vi "Lift main.vi"() -> ()   [LabVIEW 2018]
uses:
  <vilib>/Rock Robotics/WPI/ThirdParty/Phoenix-LabVIEW/Motor Controller/Controls/CTRE_Phoenix_MotorControl_FeedbackDevice.ctl
  <vilib>/Rock Robotics/WPI/ThirdParty/Phoenix-LabVIEW/Motor Controller/Controls/CTRE_Phoenix_MotorControl_ControlMode.ctl
  <vilib>/Rock Robotics/WPI/ThirdParty/Phoenix-LabVIEW/Motor Controller/Get/CTRE_Phoenix_MotorController_GetSelectedSensorData.vi
  <vilib>/Rock Robotics/Network Tables/NT Write Number.vi
  <vilib>/Rock Robotics/Network Tables/NT Read Boolean.vi
  Robot Global Data.vi
  <vilib>/Rock Robotics/Network Tables/NT Read Number.vi
  <vilib>/Rock Robotics/WPI/Solenoid/Deprecated/WPI_SolenoidSetBool.vi
panel:
  in  "Calibrate Lift":bool
  in  "Lift Setpoint":dbl
  in  "Enable Manual":bool
  in  "Disable?":bool
  in  "Lift Shift":bool
  in  "reset pos":bool
  in  "Setpoint":dbl
  in  "Output":dbl(slide) scale=-1.0..1.0
  in  "Lift Selector":enum16{"Motion Magic", "Manual", "Disable"}(ring)
  in  "PIDF":T1={"P"=2.0, "I"=0.0, "D"=0.0, "F"=0.0, "I zone"=0.0}
  out "Velocity (Raw Sensor Units per 100 ms)":i32
  out "Position (Raw Sensor Units)":i32
  in  "Acceleration":i32=2000
  in  "Cruise Velocity":i32=2000
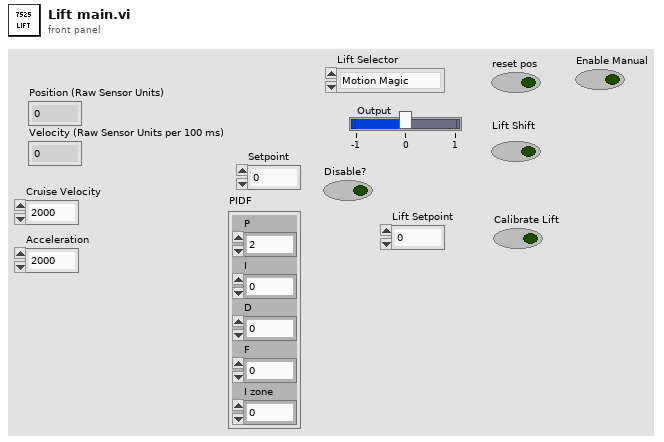
[diagram p1: front panel]
types:
  T1 = cluster{"P":dbl, "I":dbl, "D":dbl, "F":dbl, "I zone":dbl}
  T2 = enum16{"Idle", "Ground", "Hatch Low", "Hatch Mid", "Hatch High", "Cargo Low", "Cargo Mid", "Cargo High", "Cargo Ship", "Cargo Feed"}
  T3 = typedef "CTRE_Phoenix_MotorControl_FeedbackDevice.ctl" = i8
  T4 = typedef "WPI_SolenoidDevRef.ctl" = cluster{"DevStatus":errorcluster, "Pneumatics Control Module":u8, "Forward Solenoid Channel":T5, "Reverse Solenoid Channel":T5}
  T5 = typedef "WPI_SolenoidChannel.ctl" = enum8{"Solenoid 0", "Solenoid 1", "Solenoid 2", "Solenoid 3", "Solenoid 4", "Solenoid 5", "Solenoid 6", "Solenoid 7", "Invalid"}
  T6 = typedef "WPI_MotorControlDeviceRef.ctl" = cluster{"DeviceStatus":errorcluster, "Type":T7, "PWM":cluster{"PWM Channel":T8, "DeadBand":T9}, "CAN":cluster{"Device Number":u8, "SetOutput VI Ref":variant, "GetOutput VI Ref":variant, "Enable VI Ref":variant, "Disable VI Ref":variant, "Data":variant}, "Invert":bool, "DIO PWM":cluster{"PWM \"Enable\" Channel":T8, "DIOChannel":T10, "PWM Rate":dbl}}
  T7 = typedef "WPI_MotorControlType.ctl" = enum16{"PWM", "CAN", "DIO PWM"}
  T8 = typedef "FPGA_DIOPWMChannel.ctl" = enum8{"PWM 0", "PWM 1", "PWM 2", "PWM 3", "PWM 4", "PWM 5", "PWM 6", "PWM 7", "PWM 8", "PWM 9", "PWM MXP 0", "PWM MXP 1", "PWM MXP 2", "PWM MXP 3", "PWM MXP 4", "PWM MXP 5", "PWM MXP 6", "PWM MXP 7", "PWM MXP 8", "PWM MXP 9", "Invalid"}
  T9 = typedef "WPI_PWMDeadband.ctl" = cluster{"Name":string, "maxPositivePwm":i32, "minPositivePwm":i32, "centerPwm":i32, "maxNegativePwm":i32, "minNegativePwm":i32, "angularRange":u16}
  T10 = typedef "FPGA_DIOChannel.ctl" = enum8{"DIO 0", "DIO 1", "DIO 2", "DIO 3", "DIO 4", "DIO 5", "DIO 6", "DIO 7", "DIO 8", "DIO 9", "DIO MXP 0", "DIO MXP 1", "DIO MXP 2", "DIO MXP 3", "DIO MXP 4", "DIO MXP 5", "DIO MXP 6", "DIO MXP 7", "DIO MXP 8", "DIO MXP 9", "DIO MXP 10", "DIO MXP 11", "DIO MXP 12", "DIO MXP 13", "DIO MXP 14", "DIO MXP 15", "SPI Port CS1", "SPI Port CS2", "SPI Port CS3", "SPI Port MISO", "SPI Port MOSI", "Invalid"}
  T11 = enum16{"Idle", "Ground", "Hatch Low", "Hatch Mid", "Hatch High", "Cargo Low", "Cargo Mid", "Cargo High", "Cargo Ship", "Cargo Feed"}[]
  T12 = typedef "CTRE_Phoenix_MotorControl_ControlMode.ctl" = u16
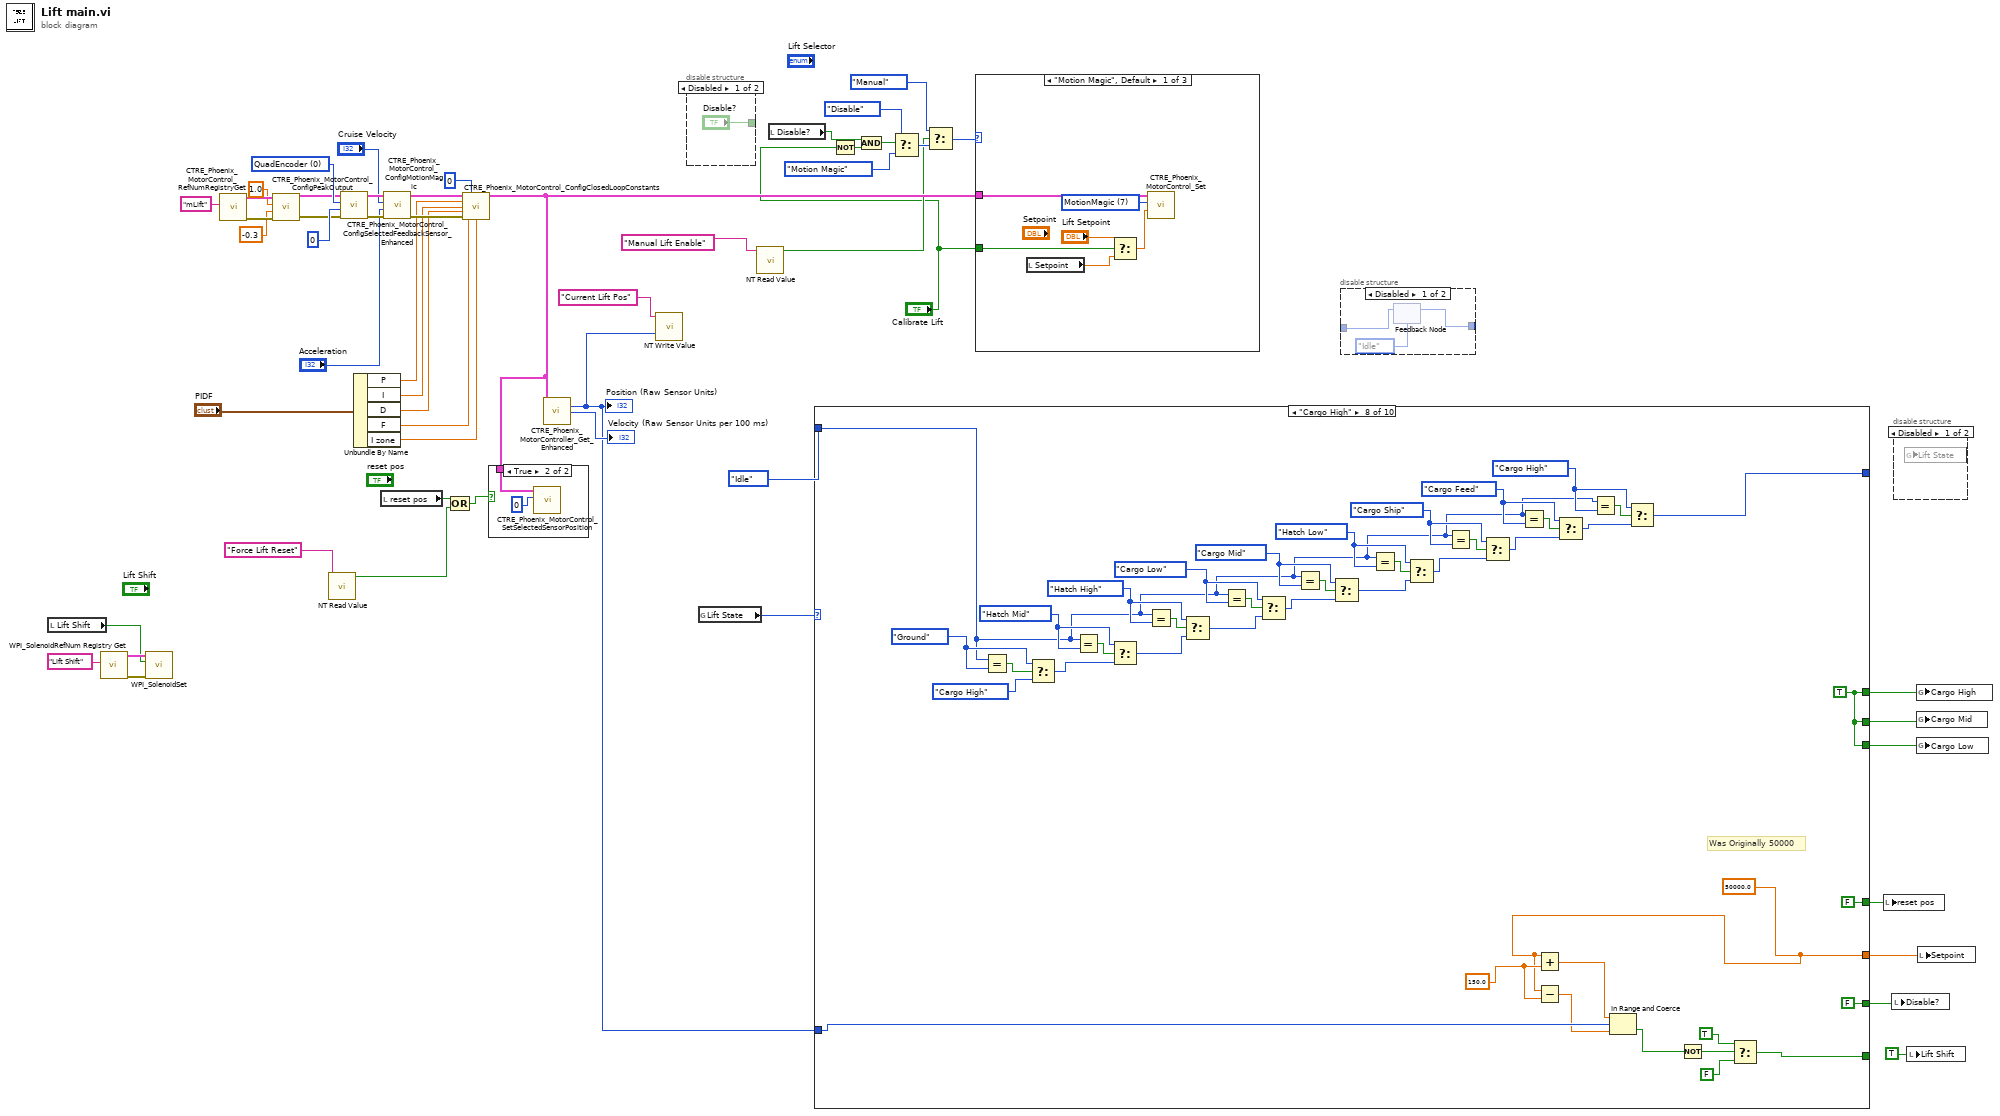
[diagram p0: block diagram]
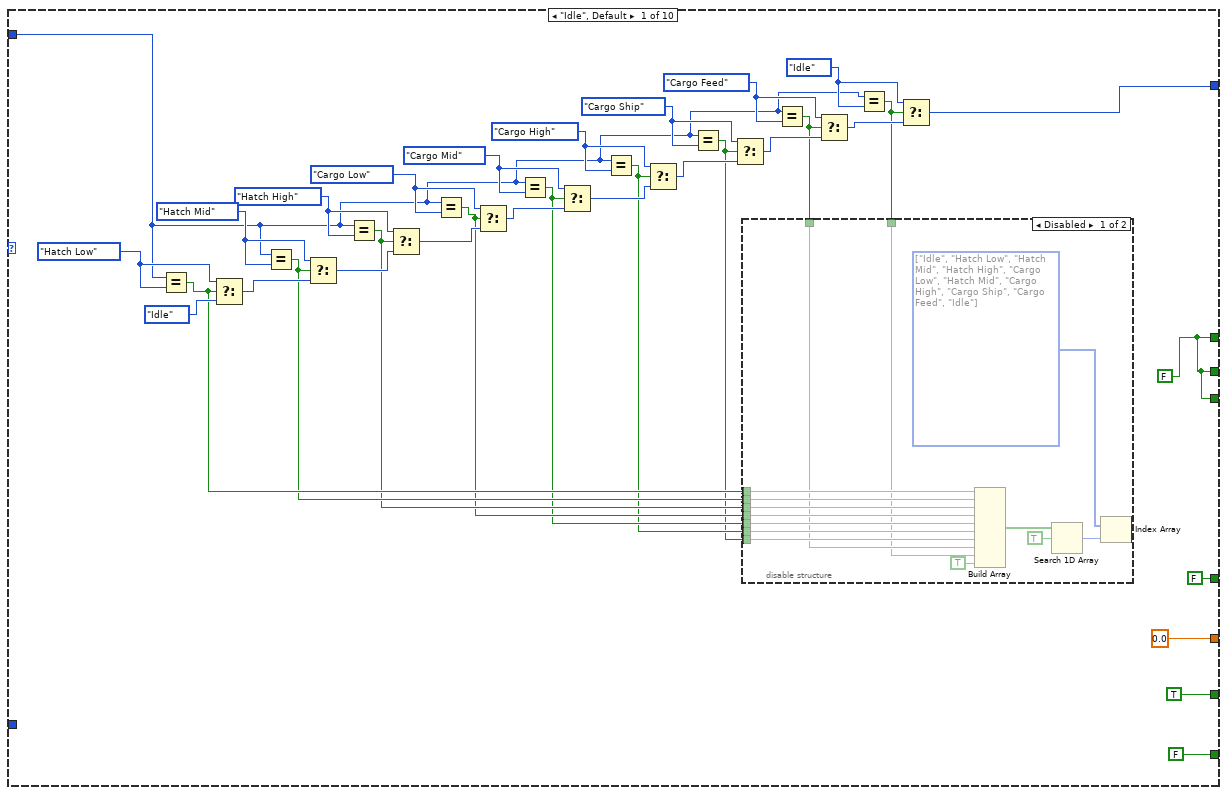
[diagram p5: hidden frame]
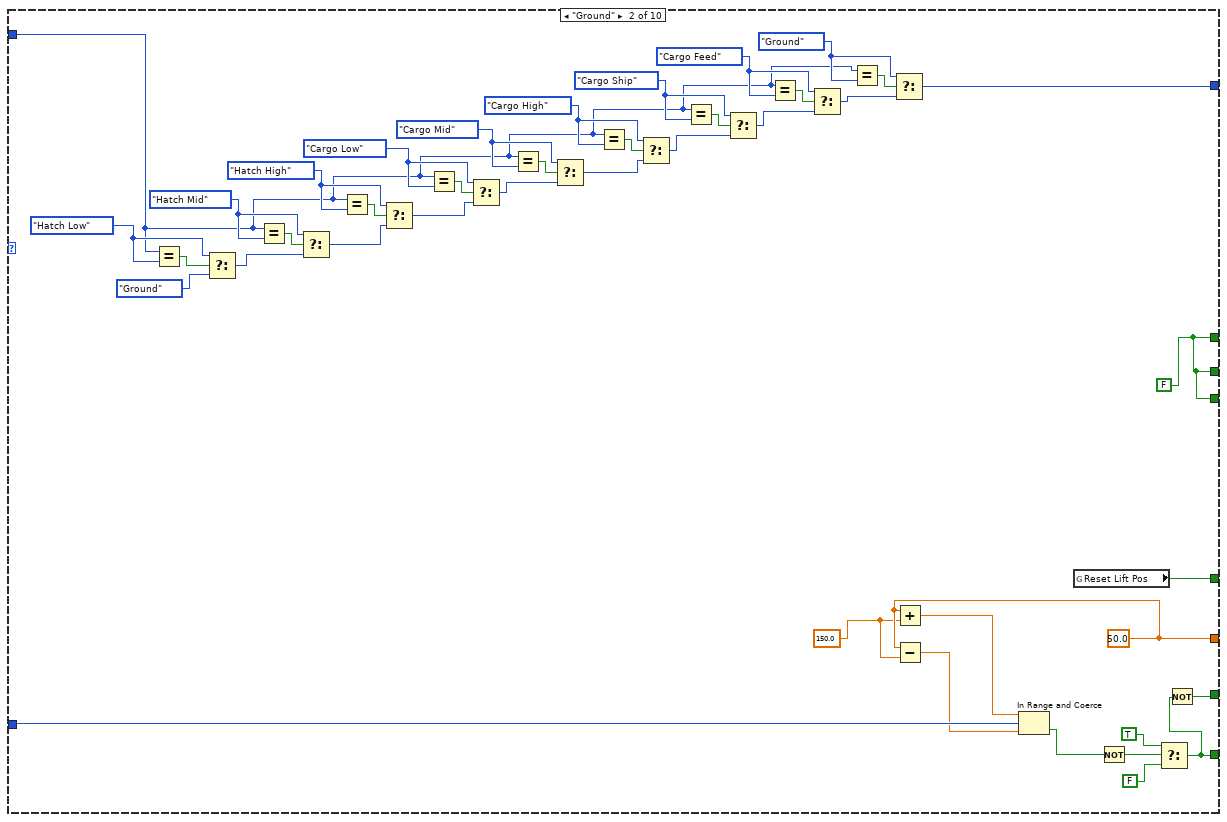
[diagram p7: hidden frame]
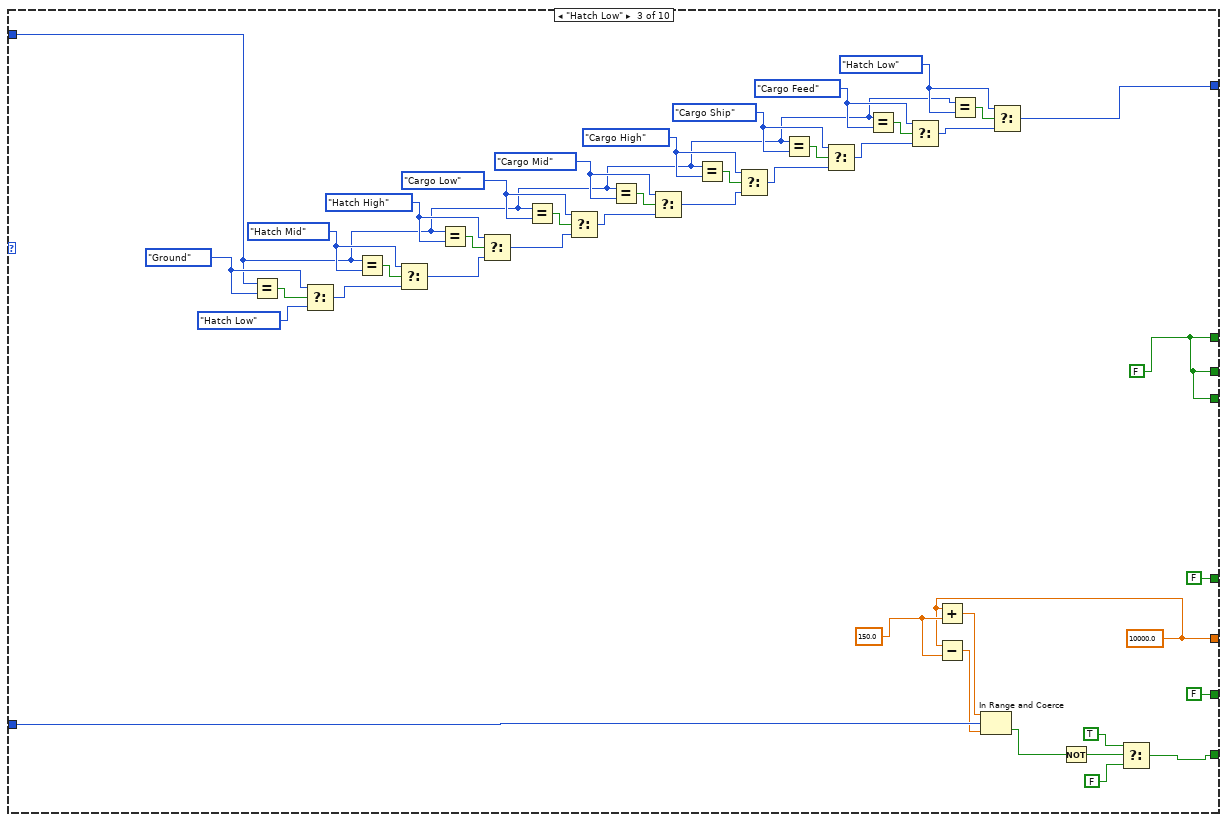
[diagram p8: hidden frame]
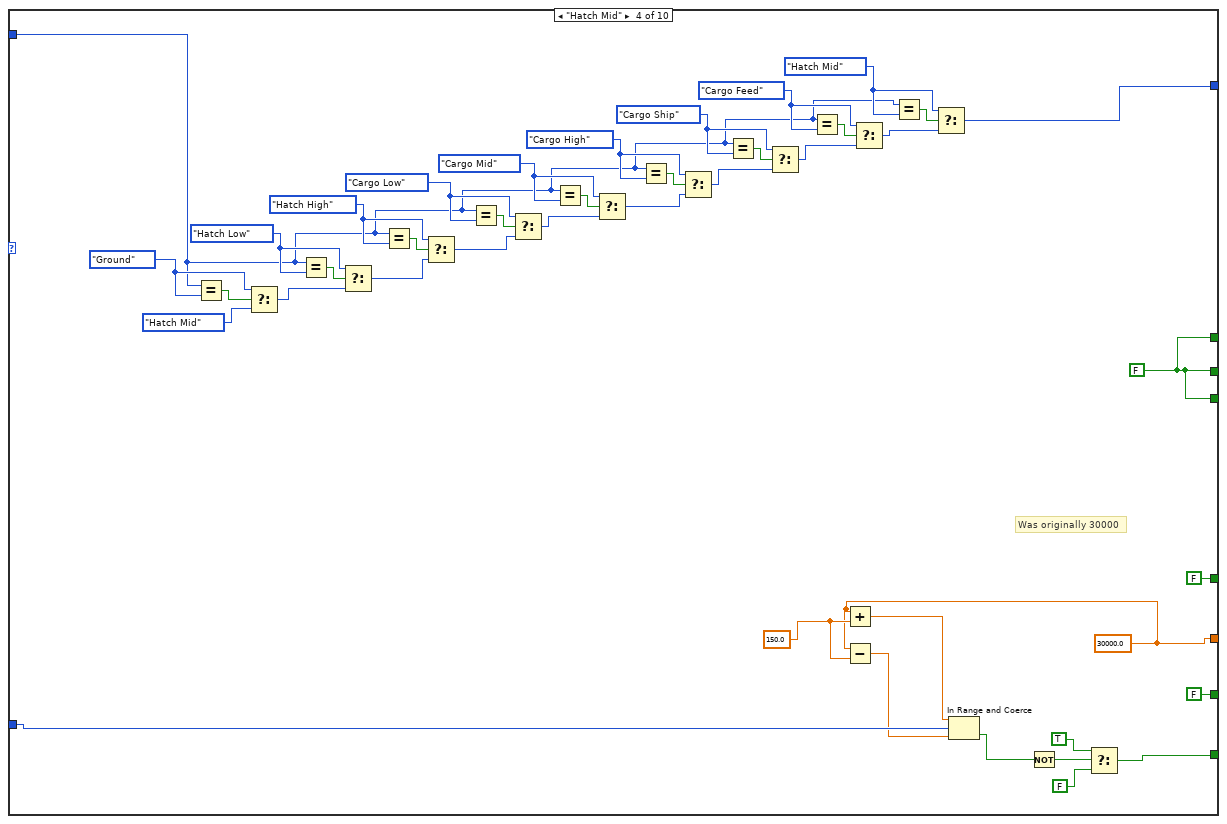
[diagram p9: hidden frame]
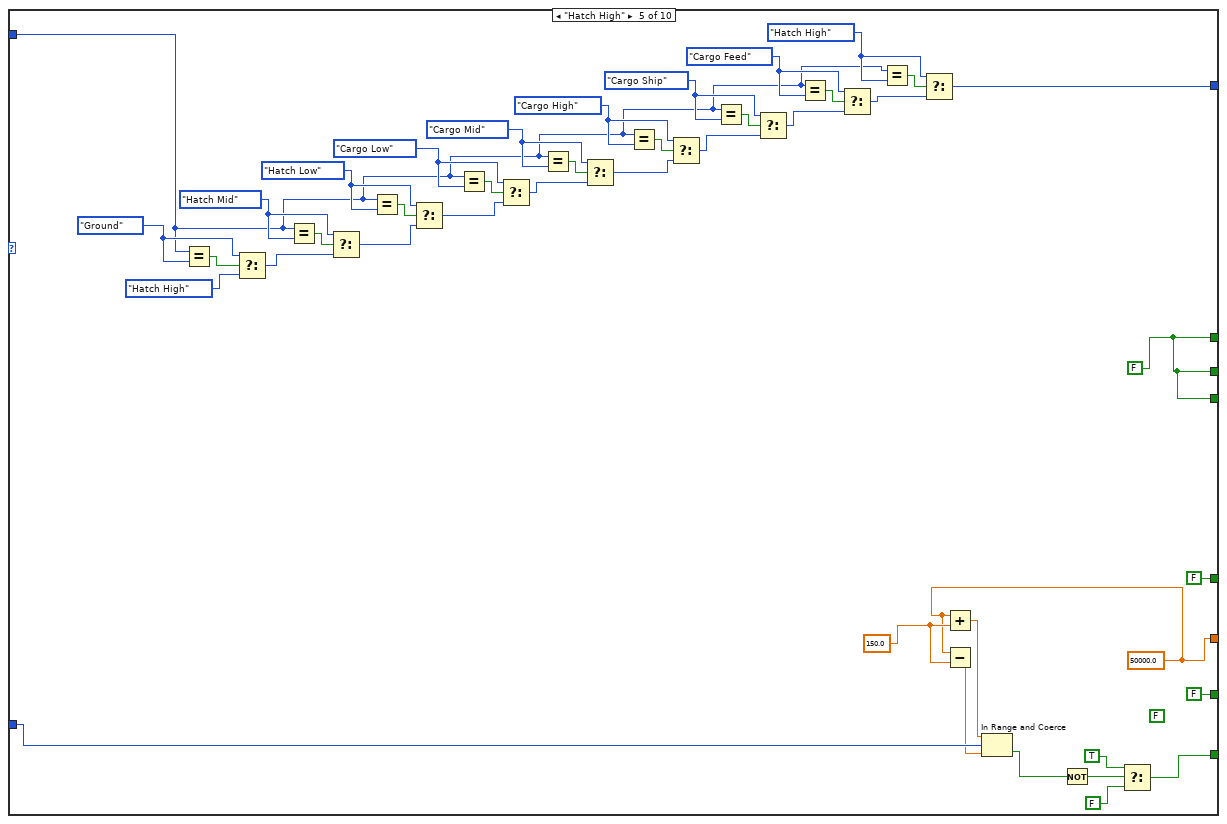
[diagram p10: hidden frame]
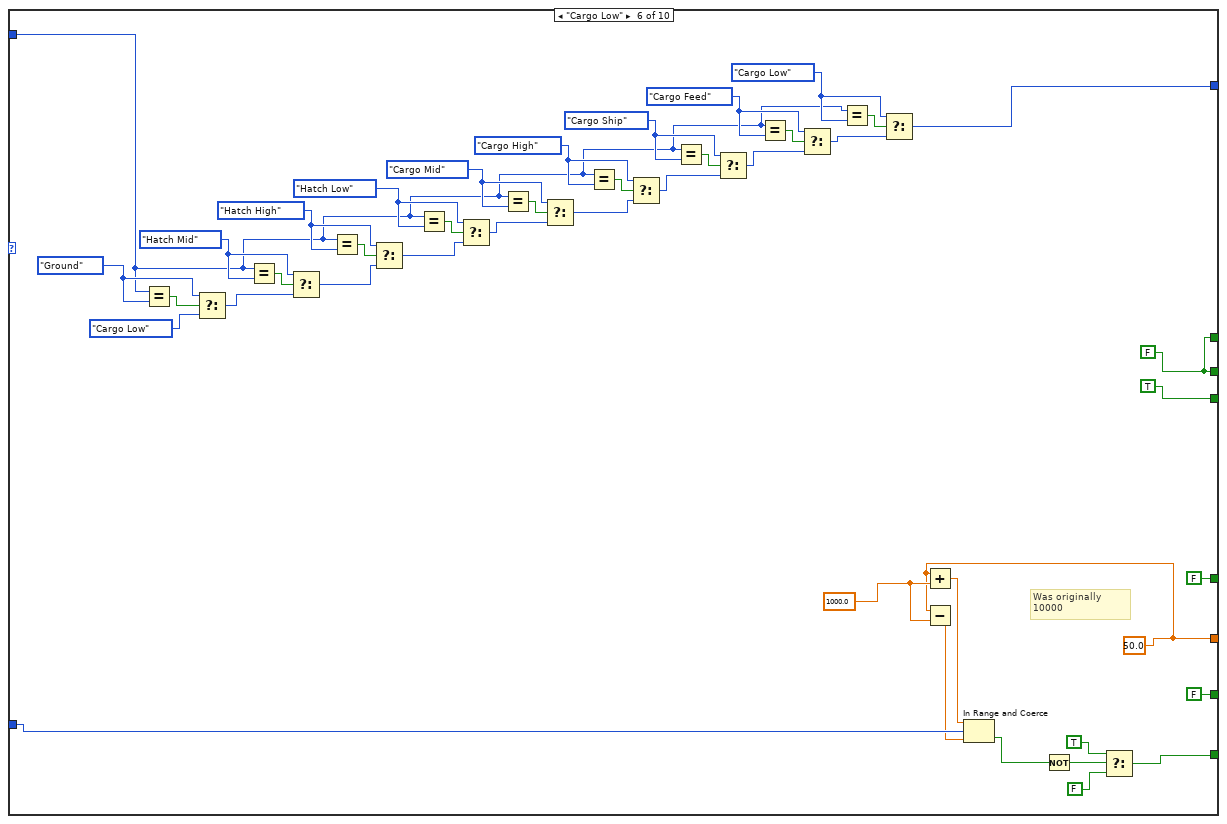
[diagram p11: hidden frame]
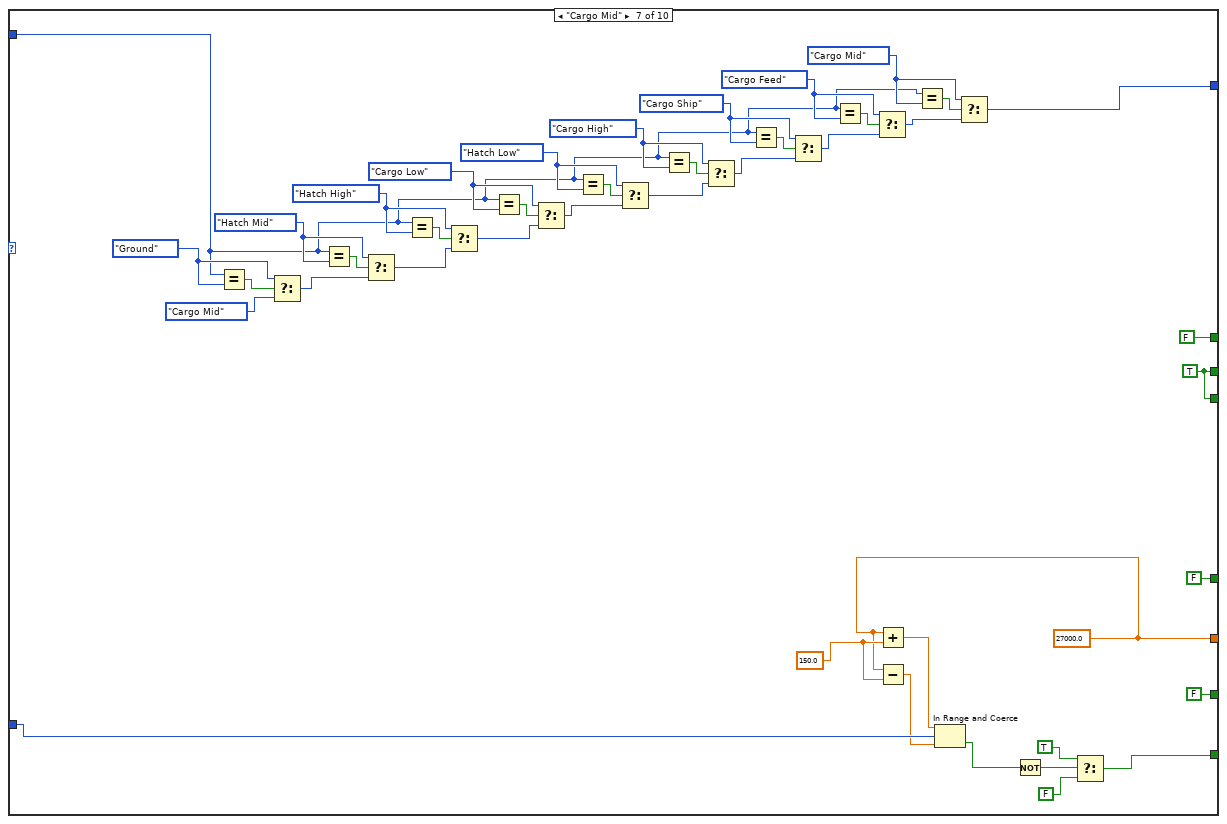
[diagram p12: hidden frame]
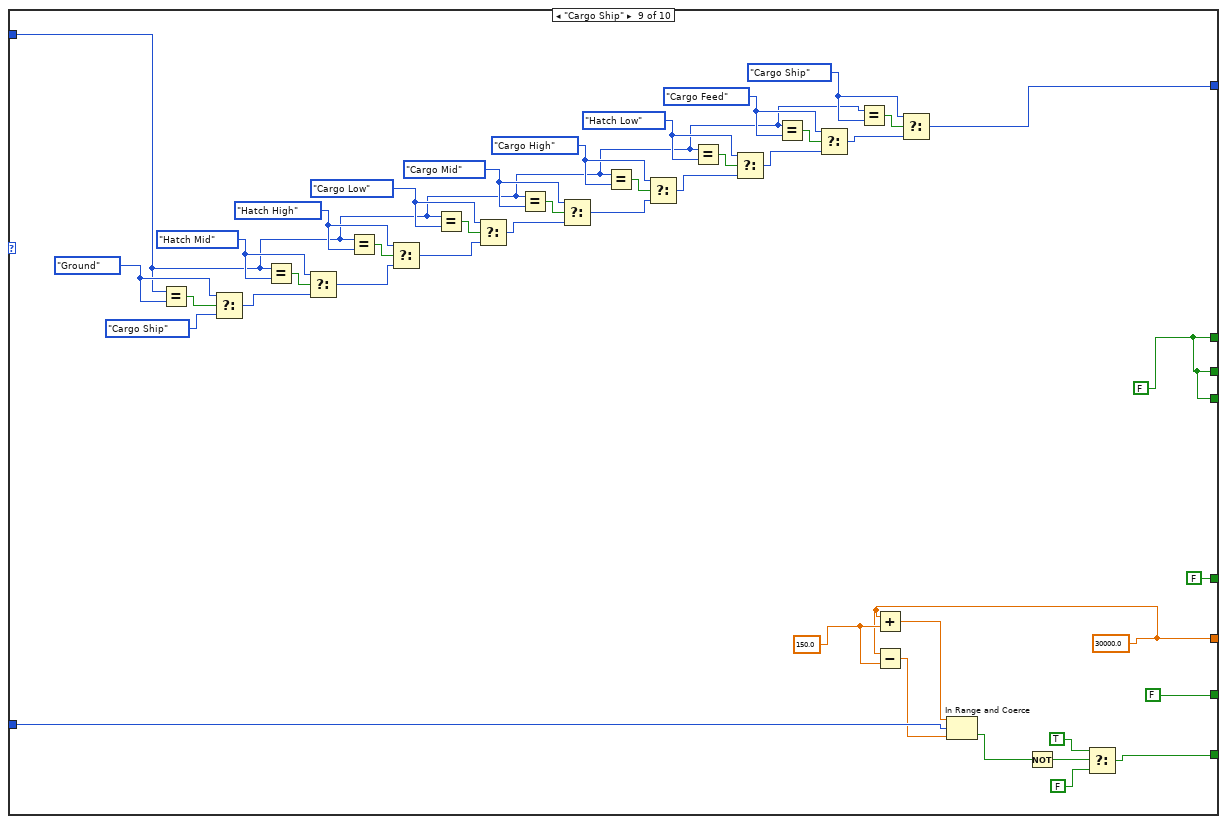
[diagram p13: hidden frame]
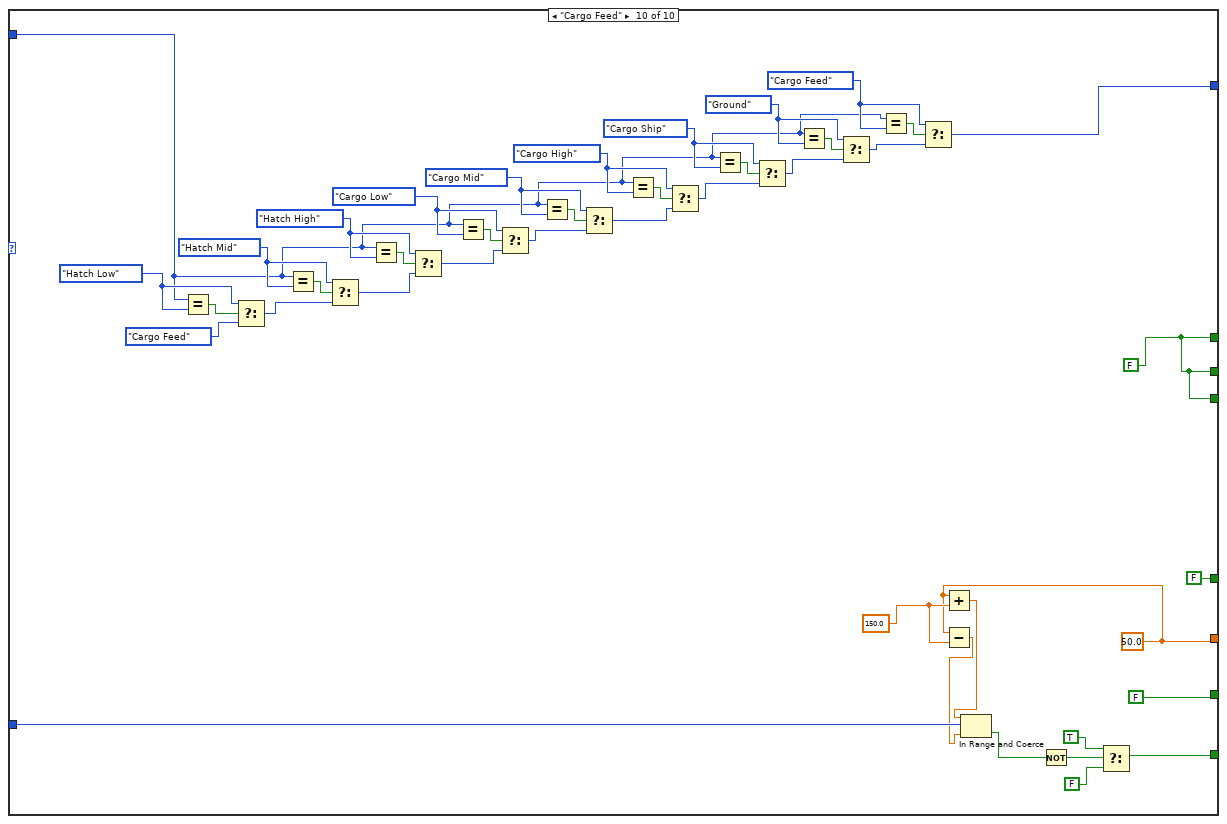
[diagram p14: hidden frame]
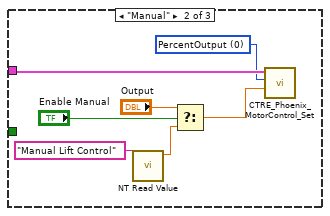
[diagram p16: hidden frame]
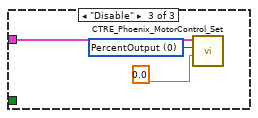
[diagram p17: hidden frame]
diagram:
  w49 = T3 0 items=["QuadEncoder"=0, "Analog"=2, "Tachometer"=4, "Pulse Width Encoded Position"=8, "Sensor Sum (S0 + S1)"=9, "Sensor Difference (D0 - D1)"=10, "Remote Source 0"=11, "Remote Source 1"=12, "Software Emulated"=15] ("Feedback Device")
  n1 = local read "Lift Shift"() -> (w24:bool)
  n2 = call <vilib>:"WPI_SolenoidRefNum Registry Get.vi"("refnum name"="Lift Shift") -> ("error out"=w30:errorcluster, "SolenoidDevRef"=w29:T4)  [unwired: 9 in]
  n3 = call-poly <vilib>:"WPI_SolenoidSet.vi"("error in (no error)"=w30, "Value"=w24, "SolenoidDevRef"=w29) -> ()  [unwired: 7 in, 2 out]
  n4 = call <vilib>:"CTRE_Phoenix_MotorControl_RefNumRegistryGet.vi"("refnum name"="mLift") -> ("error out"=w53:errorcluster, "PhoenixMotorControlDevRef"=w52:T6)  [unwired: 9 in]
  n5 = call <vilib>:"CTRE_Phoenix_MotorControl_ConfigPeakOutput.vi"("error in (no error)"=w53, "Reverse Peak Percent Output"=-0.3, "Forward Peak Percent Output"=1.0, "PhoenixMotorControlDevRef"=w52) -> ("error out"=w46:errorcluster, "PhoenixMotorControlDevRef"=w47:T6)  [unwired: 6 in]
  n6 = call-poly <vilib>:"NT Read Value.vi"("Name"="Force Lift Reset") -> ("Boolean"=w9:bool)  [unwired: 9 in, 1 out]
  n7 = call <vilib>:"CTRE_Phoenix_MotorControl_ConfigSelectedFeedbackSensor_Enhanced.vi"("error in (no error)"=w46, "pidLoopIdx"=0, "Feedback Device"=w49, "PhoenixMotorControlDevRef"=w47) -> ("error out"=w45:errorcluster, "PhoenixMotorControlDevRef"=w44:T6)  [unwired: 6 in]
  n8 = Unbundle By Name("PIDF") -> ("P"=w36:dbl, "I"=w35:dbl, "D"=w34:dbl, "F"=w33:dbl, "I zone"=w32:dbl)
  n9 = local read "reset pos"() -> (w10:bool)
  n10 = call <vilib>:"CTRE_Phoenix_MotorControl_ConfigMotionMagic.vi"("error in (no error)"=w45, "Acceleration"="Acceleration", "Cruise Velocity"="Cruise Velocity", "PhoenixMotorControlDevRef"=w44) -> ("error out"=w39:errorcluster, "PhoenixMotorControlDevRef"=w40:T6)  [unwired: 6 in]
  n11 = Or(x=w10, y=w9) -> (x .or. y?=w11:bool)
  n12 = call <vilib>:"CTRE_Phoenix_MotorControl_ConfigClosedLoopConstants.vi"("PhoenixMotorControlDevRef"=w40, "slotIdx"=0, "P"=w36, "I"=w35, "D"=w34, "error in (no error)"=w39, "F"=w33, "I Zone"=w32) -> ("PhoenixMotorControlDevRef"=w31:T6)  [unwired: 6 in, 1 out]
  n13 = case shown="True" w11 {
    tunnel: w31 -> [_ w56]
    frame False {
    }
    frame True {
      n14 = call <vilib>:"CTRE_Phoenix_MotorControl_SetSelectedSensorPosition.vi"("New Sensor Position"=0, "PhoenixMotorControlDevRef"=w56) -> ()  [unwired: 8 in, 2 out]
    }
  }
  n15 = call-poly <vilib>:"CTRE_Phoenix_MotorController_Get_Enhanced.vi"("PhoenixMotorControlDevRef"=w31) -> ("Position (Raw Sensor Units)"=w20:i32, "Velocity (Raw Sensor Units per 100 ms)"=→"Velocity (Raw Sensor Units per 100 ms)":i32)  [unwired: 11 in, 2 out]
  "Position (Raw Sensor Units)" <- w20
  n16 = call-poly <vilib>:"NT Write Value.vi"("Numeric"=w20, "Name"="Current Lift Pos") -> ()  [unwired: 9 in, 1 out]
  n17 = disable-structure shown="Disabled" {
    disable-tunnel: ["Disable?" _] -> _
    frame Disabled {
    }
    frame Enabled {
    }
  }
  n18 = global read "Robot Global Data.vi" "Lift State"() -> (w12:T2)
  n19 = call-poly <vilib>:"NT Read Value.vi"("Name"="Manual Lift Enable") -> ("Boolean"=w14:bool)  [unwired: 9 in, 1 out]
  n20 = local read "Disable?"() -> (w4:bool)
  n21 = case shown="\"Cargo High\"" w12 {
    tunnel: T2."Idle" ("Lift State") -> [w73 w120 w162 w204 w246 w289 w332 w374 w416 w458]
    tunnel: [w72 w119 w161 w203 w245 w288 w331 w373 w415 w457] -> _
    tunnel: [TRUE w112 FALSE FALSE FALSE FALSE FALSE FALSE FALSE FALSE] -> w26
    tunnel: [0.0 w110 w151 w191 w235 w278 w321 w361 w405 w445] -> w25
    tunnel: [FALSE w111 w155 w197 w239 w282 w324 w366 w408 w449] -> _
    tunnel: [FALSE ("Reset Lift Pos") w118 FALSE ("Reset Lift Pos") FALSE ("Reset Lift Pos") FALSE ("Reset Lift Pos") FALSE ("Reset Lift Pos") FALSE ("Reset Lift Pos") FALSE ("Reset Lift Pos") FALSE ("Reset Lift Pos") FALSE ("Reset Lift Pos")] -> w23
    tunnel: w20 -> [_ w113 w154 w196 w238 w281 w325 w365 w407 w452]
    tunnel: [w58 w106 w148 w190 w232 w274 FALSE w360 w402 w444] -> w7
    tunnel: [w58 w106 w148 w190 w232 w274 w317 w360 w402 w444] -> w6
    tunnel: [w58 w106 w148 w190 w232 TRUE w317 w360 w402 w444] -> w5
    frame "Idle", Default {
      w58 = FALSE
      w75 = T2."Idle" ("Lift State")
      w77 = T2."Cargo Feed" ("Lift State")
      w79 = T2."Cargo Ship" ("Lift State")
      w81 = T2."Cargo High" ("Lift State")
      w83 = T2."Cargo Mid" ("Lift State")
      w85 = T2."Cargo Low" ("Lift State")
      w87 = T2."Hatch High" ("Lift State")
      w89 = T2."Hatch Mid" ("Lift State")
      w90 = T2."Hatch Low" ("Lift State")
      n22 = Equal?(x=w73, y=w90) -> (x = y?=w71:bool)
      n23 = Select(t=w90, s=w71, f=T2."Idle" ("Lift State")) -> (s? t:f=w88:T2)
      n24 = Equal?(x=w73, y=w89) -> (x = y?=w70:bool)
      n25 = Select(t=w89, s=w70, f=w88) -> (s? t:f=w86:T2)
      n26 = Equal?(x=w73, y=w87) -> (x = y?=w69:bool)
      n27 = Select(t=w87, s=w69, f=w86) -> (s? t:f=w84:T2)
      n28 = Equal?(x=w73, y=w85) -> (x = y?=w68:bool)
      n29 = Select(t=w85, s=w68, f=w84) -> (s? t:f=w82:T2)
      n30 = Equal?(x=w73, y=w83) -> (x = y?=w67:bool)
      n31 = Select(t=w83, s=w67, f=w82) -> (s? t:f=w80:T2)
      n32 = Equal?(x=w73, y=w81) -> (x = y?=w66:bool)
      n33 = Select(t=w81, s=w66, f=w80) -> (s? t:f=w78:T2)
      n34 = Equal?(x=w73, y=w79) -> (x = y?=w65:bool)
      n35 = Select(t=w79, s=w65, f=w78) -> (s? t:f=w76:T2)
      n36 = Equal?(x=w73, y=w77) -> (x = y?=w64:bool)
      n37 = Select(t=w77, s=w64, f=w76) -> (s? t:f=w74:T2)
      n38 = Equal?(x=w73, y=w75) -> (x = y?=w63:bool)
      n39 = disable-structure shown="Disabled" {
        disable-tunnel: w71 -> [w105 _]
        disable-tunnel: w70 -> [w104 _]
        disable-tunnel: w69 -> [w103 _]
        disable-tunnel: w68 -> [w102 _]
        disable-tunnel: w67 -> [w101 _]
        disable-tunnel: w66 -> [w100 _]
        disable-tunnel: w65 -> [w99 _]
        disable-tunnel: w64 -> [w98 _]
        disable-tunnel: w63 -> [w97 _]
        frame Disabled {
          w92 = T11 [enum."Idle", enum."Hatch Low", enum."Hatch Mid", enum."Hatch High", enum."Cargo Low", enum."Hatch Mid", enum."Cargo High", enum."Cargo Ship", enum."Cargo Feed", enum."Idle"] items=["Idle", "Ground", "Hatch Low", "Hatch Mid", "Hatch High", "Cargo Low", "Cargo Mid", "Cargo High", "Cargo Ship", "Cargo Feed"]
          n40 = Build Array(w105, w104, w103, w102, w101, w100, w99, w98, w97, TRUE ("element")) -> (w95:bool[])
          n41 = Search 1D Array(1D array=w95, element=TRUE) -> (index of element=w93:i32)  [unwired: 1 in]
          n42 = Index Array(array=w92, index=w93) -> ()  [unwired: 1 out]
        }
        frame Enabled {
        }
      }
      n43 = Select(t=w75, s=w63, f=w74) -> (s? t:f=w72:T2)
    }
    frame "Ground" {
      w106 = FALSE
      w109 = 150.0
      w110 = 50.0
      w123 = T2."Ground" ("Lift State")
      w126 = T2."Cargo Feed" ("Lift State")
      w129 = T2."Cargo Ship" ("Lift State")
      w132 = T2."Cargo High" ("Lift State")
      w135 = T2."Cargo Mid" ("Lift State")
      w138 = T2."Cargo Low" ("Lift State")
      w141 = T2."Hatch High" ("Lift State")
      w144 = T2."Hatch Mid" ("Lift State")
      w145 = T2."Hatch Low" ("Lift State")
      n44 = Equal?(x=w120, y=w145) -> (x = y?=w146:bool)
      n45 = Select(t=w145, s=w146, f=T2."Ground" ("Lift State")) -> (s? t:f=w142:T2)
      n46 = Equal?(x=w120, y=w144) -> (x = y?=w143:bool)
      n47 = Select(t=w144, s=w143, f=w142) -> (s? t:f=w139:T2)
      n48 = Equal?(x=w120, y=w141) -> (x = y?=w140:bool)
      n49 = Select(t=w141, s=w140, f=w139) -> (s? t:f=w136:T2)
      n50 = Equal?(x=w120, y=w138) -> (x = y?=w137:bool)
      n51 = Select(t=w138, s=w137, f=w136) -> (s? t:f=w133:T2)
      n52 = Equal?(x=w120, y=w135) -> (x = y?=w134:bool)
      n53 = Select(t=w135, s=w134, f=w133) -> (s? t:f=w130:T2)
      n54 = Equal?(x=w120, y=w132) -> (x = y?=w131:bool)
      n55 = Select(t=w132, s=w131, f=w130) -> (s? t:f=w127:T2)
      n56 = Equal?(x=w120, y=w129) -> (x = y?=w128:bool)
      n57 = Select(t=w129, s=w128, f=w127) -> (s? t:f=w124:T2)
      n58 = Equal?(x=w120, y=w126) -> (x = y?=w125:bool)
      n59 = Select(t=w126, s=w125, f=w124) -> (s? t:f=w121:T2)
      n60 = Equal?(x=w120, y=w123) -> (x = y?=w122:bool)
      n61 = Select(t=w123, s=w122, f=w121) -> (s? t:f=w119:T2)
      n62 = Add(x=w110, y=w109) -> (x+y=w107:dbl)
      n63 = Subtract(x=w110, y=w109) -> (x-y=w108:dbl)
      n64 = In Range and Coerce(upper limit=w107, x=w113, lower limit=w108) -> (In Range?=w115:bool)  [unwired: 1 out]
      n65 = global read "Robot Global Data.vi" "Reset Lift Pos"() -> (w118:bool)
      n66 = Not(x=w115) -> (.not. x?=w114:bool)
      n67 = Select(t=TRUE, s=w114, f=FALSE) -> (s? t:f=w111:bool)
      n68 = Not(x=w111) -> (.not. x?=w112:bool)
    }
    frame "Hatch Low" {
      w148 = FALSE
      w152 = 150.0
      w151 = 10000.0
      w165 = T2."Hatch Low" ("Lift State")
      w168 = T2."Cargo Feed" ("Lift State")
      w171 = T2."Cargo Ship" ("Lift State")
      w174 = T2."Cargo High" ("Lift State")
      w177 = T2."Cargo Mid" ("Lift State")
      w180 = T2."Cargo Low" ("Lift State")
      w183 = T2."Hatch High" ("Lift State")
      w186 = T2."Hatch Mid" ("Lift State")
      w187 = T2."Ground" ("Lift State")
      n69 = Equal?(x=w162, y=w187) -> (x = y?=w188:bool)
      n70 = Select(t=w187, s=w188, f=T2."Hatch Low" ("Lift State")) -> (s? t:f=w184:T2)
      n71 = Equal?(x=w162, y=w186) -> (x = y?=w185:bool)
      n72 = Select(t=w186, s=w185, f=w184) -> (s? t:f=w181:T2)
      n73 = Equal?(x=w162, y=w183) -> (x = y?=w182:bool)
      n74 = Select(t=w183, s=w182, f=w181) -> (s? t:f=w178:T2)
      n75 = Equal?(x=w162, y=w180) -> (x = y?=w179:bool)
      n76 = Select(t=w180, s=w179, f=w178) -> (s? t:f=w175:T2)
      n77 = Equal?(x=w162, y=w177) -> (x = y?=w176:bool)
      n78 = Select(t=w177, s=w176, f=w175) -> (s? t:f=w172:T2)
      n79 = Equal?(x=w162, y=w174) -> (x = y?=w173:bool)
      n80 = Select(t=w174, s=w173, f=w172) -> (s? t:f=w169:T2)
      n81 = Equal?(x=w162, y=w171) -> (x = y?=w170:bool)
      n82 = Select(t=w171, s=w170, f=w169) -> (s? t:f=w166:T2)
      n83 = Equal?(x=w162, y=w168) -> (x = y?=w167:bool)
      n84 = Select(t=w168, s=w167, f=w166) -> (s? t:f=w163:T2)
      n85 = Add(x=w151, y=w152) -> (x+y=w150:dbl)
      n86 = Subtract(x=w151, y=w152) -> (x-y=w149:dbl)
      n87 = Equal?(x=w162, y=w165) -> (x = y?=w164:bool)
      n88 = In Range and Coerce(upper limit=w150, x=w154, lower limit=w149) -> (In Range?=w157:bool)  [unwired: 1 out]
      n89 = Select(t=w165, s=w164, f=w163) -> (s? t:f=w161:T2)
      n90 = Not(x=w157) -> (.not. x?=w156:bool)
      n91 = Select(t=TRUE, s=w156, f=FALSE) -> (s? t:f=w155:bool)
    }
    frame "Hatch Mid" {
      w190 = FALSE
      w194 = 150.0
      w191 = 30000.0
      w207 = T2."Hatch Mid" ("Lift State")
      w210 = T2."Cargo Feed" ("Lift State")
      w213 = T2."Cargo Ship" ("Lift State")
      w216 = T2."Cargo High" ("Lift State")
      w219 = T2."Cargo Mid" ("Lift State")
      w222 = T2."Cargo Low" ("Lift State")
      w225 = T2."Hatch High" ("Lift State")
      w228 = T2."Hatch Low" ("Lift State")
      w229 = T2."Ground" ("Lift State")
      # "Was originally 30000"
      n92 = Equal?(x=w204, y=w229) -> (x = y?=w230:bool)
      n93 = Select(t=w229, s=w230, f=T2."Hatch Mid" ("Lift State")) -> (s? t:f=w226:T2)
      n94 = Equal?(x=w204, y=w228) -> (x = y?=w227:bool)
      n95 = Select(t=w228, s=w227, f=w226) -> (s? t:f=w223:T2)
      n96 = Equal?(x=w204, y=w225) -> (x = y?=w224:bool)
      n97 = Select(t=w225, s=w224, f=w223) -> (s? t:f=w220:T2)
      n98 = Equal?(x=w204, y=w222) -> (x = y?=w221:bool)
      n99 = Select(t=w222, s=w221, f=w220) -> (s? t:f=w217:T2)
      n100 = Equal?(x=w204, y=w219) -> (x = y?=w218:bool)
      n101 = Select(t=w219, s=w218, f=w217) -> (s? t:f=w214:T2)
      n102 = Equal?(x=w204, y=w216) -> (x = y?=w215:bool)
      n103 = Select(t=w216, s=w215, f=w214) -> (s? t:f=w211:T2)
      n104 = Equal?(x=w204, y=w213) -> (x = y?=w212:bool)
      n105 = Select(t=w213, s=w212, f=w211) -> (s? t:f=w208:T2)
      n106 = Equal?(x=w204, y=w210) -> (x = y?=w209:bool)
      n107 = Add(x=w191, y=w194) -> (x+y=w192:dbl)
      n108 = Subtract(x=w191, y=w194) -> (x-y=w193:dbl)
      n109 = Select(t=w210, s=w209, f=w208) -> (s? t:f=w205:T2)
      n110 = Equal?(x=w204, y=w207) -> (x = y?=w206:bool)
      n111 = Select(t=w207, s=w206, f=w205) -> (s? t:f=w203:T2)
      n112 = In Range and Coerce(upper limit=w192, x=w196, lower limit=w193) -> (In Range?=w199:bool)  [unwired: 1 out]
      n113 = Not(x=w199) -> (.not. x?=w198:bool)
      n114 = Select(t=TRUE, s=w198, f=FALSE) -> (s? t:f=w197:bool)
    }
    frame "Hatch High" {
      w232 = FALSE
      w236 = 150.0
      w235 = 50000.0
      (unwired) FALSE
      w249 = T2."Hatch High" ("Lift State")
      w252 = T2."Cargo Feed" ("Lift State")
      w255 = T2."Cargo Ship" ("Lift State")
      w258 = T2."Cargo High" ("Lift State")
      w261 = T2."Cargo Mid" ("Lift State")
      w264 = T2."Cargo Low" ("Lift State")
      w267 = T2."Hatch Low" ("Lift State")
      w270 = T2."Hatch Mid" ("Lift State")
      w271 = T2."Ground" ("Lift State")
      n115 = Equal?(x=w246, y=w271) -> (x = y?=w272:bool)
      n116 = Select(t=w271, s=w272, f=T2."Hatch High" ("Lift State")) -> (s? t:f=w268:T2)
      n117 = Equal?(x=w246, y=w270) -> (x = y?=w269:bool)
      n118 = Select(t=w270, s=w269, f=w268) -> (s? t:f=w265:T2)
      n119 = Equal?(x=w246, y=w267) -> (x = y?=w266:bool)
      n120 = Select(t=w267, s=w266, f=w265) -> (s? t:f=w262:T2)
      n121 = Equal?(x=w246, y=w264) -> (x = y?=w263:bool)
      n122 = Select(t=w264, s=w263, f=w262) -> (s? t:f=w259:T2)
      n123 = Equal?(x=w246, y=w261) -> (x = y?=w260:bool)
      n124 = Select(t=w261, s=w260, f=w259) -> (s? t:f=w256:T2)
      n125 = Equal?(x=w246, y=w258) -> (x = y?=w257:bool)
      n126 = Select(t=w258, s=w257, f=w256) -> (s? t:f=w253:T2)
      n127 = Equal?(x=w246, y=w255) -> (x = y?=w254:bool)
      n128 = Select(t=w255, s=w254, f=w253) -> (s? t:f=w250:T2)
      n129 = Equal?(x=w246, y=w252) -> (x = y?=w251:bool)
      n130 = Select(t=w252, s=w251, f=w250) -> (s? t:f=w247:T2)
      n131 = Equal?(x=w246, y=w249) -> (x = y?=w248:bool)
      n132 = Select(t=w249, s=w248, f=w247) -> (s? t:f=w245:T2)
      n133 = Add(x=w235, y=w236) -> (x+y=w234:dbl)
      n134 = Subtract(x=w235, y=w236) -> (x-y=w233:dbl)
      n135 = In Range and Coerce(upper limit=w234, x=w238, lower limit=w233) -> (In Range?=w241:bool)  [unwired: 1 out]
      n136 = Not(x=w241) -> (.not. x?=w240:bool)
      n137 = Select(t=TRUE, s=w240, f=FALSE) -> (s? t:f=w239:bool)
    }
    frame "Cargo Low" {
      w274 = FALSE
      w279 = 1000.0
      w278 = 50.0
      w292 = T2."Cargo Low" ("Lift State")
      w295 = T2."Cargo Feed" ("Lift State")
      w298 = T2."Cargo Ship" ("Lift State")
      w301 = T2."Cargo High" ("Lift State")
      w304 = T2."Cargo Mid" ("Lift State")
      w307 = T2."Hatch Low" ("Lift State")
      w310 = T2."Hatch High" ("Lift State")
      w313 = T2."Hatch Mid" ("Lift State")
      w314 = T2."Ground" ("Lift State")
      # "Was originally 10000"
      n138 = Equal?(x=w289, y=w314) -> (x = y?=w315:bool)
      n139 = Select(t=w314, s=w315, f=T2."Cargo Low" ("Lift State")) -> (s? t:f=w311:T2)
      n140 = Equal?(x=w289, y=w313) -> (x = y?=w312:bool)
      n141 = Select(t=w313, s=w312, f=w311) -> (s? t:f=w308:T2)
      n142 = Equal?(x=w289, y=w310) -> (x = y?=w309:bool)
      n143 = Select(t=w310, s=w309, f=w308) -> (s? t:f=w305:T2)
      n144 = Equal?(x=w289, y=w307) -> (x = y?=w306:bool)
      n145 = Select(t=w307, s=w306, f=w305) -> (s? t:f=w302:T2)
      n146 = Equal?(x=w289, y=w304) -> (x = y?=w303:bool)
      n147 = Select(t=w304, s=w303, f=w302) -> (s? t:f=w299:T2)
      n148 = Equal?(x=w289, y=w301) -> (x = y?=w300:bool)
      n149 = Select(t=w301, s=w300, f=w299) -> (s? t:f=w296:T2)
      n150 = Equal?(x=w289, y=w298) -> (x = y?=w297:bool)
      n151 = Select(t=w298, s=w297, f=w296) -> (s? t:f=w293:T2)
      n152 = Equal?(x=w289, y=w295) -> (x = y?=w294:bool)
      n153 = Select(t=w295, s=w294, f=w293) -> (s? t:f=w290:T2)
      n154 = Equal?(x=w289, y=w292) -> (x = y?=w291:bool)
      n155 = Select(t=w292, s=w291, f=w290) -> (s? t:f=w288:T2)
      n156 = Add(x=w278, y=w279) -> (x+y=w277:dbl)
      n157 = Subtract(x=w278, y=w279) -> (x-y=w276:dbl)
      n158 = In Range and Coerce(upper limit=w277, x=w281, lower limit=w276) -> (In Range?=w284:bool)  [unwired: 1 out]
      n159 = Not(x=w284) -> (.not. x?=w283:bool)
      n160 = Select(t=TRUE, s=w283, f=FALSE) -> (s? t:f=w282:bool)
    }
    frame "Cargo Mid" {
      w317 = TRUE
      w322 = 150.0
      w321 = 27000.0
      w335 = T2."Cargo Mid" ("Lift State")
      w338 = T2."Cargo Feed" ("Lift State")
      w341 = T2."Cargo Ship" ("Lift State")
      w344 = T2."Cargo High" ("Lift State")
      w347 = T2."Hatch Low" ("Lift State")
      w350 = T2."Cargo Low" ("Lift State")
      w353 = T2."Hatch High" ("Lift State")
      w356 = T2."Hatch Mid" ("Lift State")
      w357 = T2."Ground" ("Lift State")
      n161 = Equal?(x=w332, y=w357) -> (x = y?=w358:bool)
      n162 = Select(t=w357, s=w358, f=T2."Cargo Mid" ("Lift State")) -> (s? t:f=w354:T2)
      n163 = Equal?(x=w332, y=w356) -> (x = y?=w355:bool)
      n164 = Select(t=w356, s=w355, f=w354) -> (s? t:f=w351:T2)
      n165 = Equal?(x=w332, y=w353) -> (x = y?=w352:bool)
      n166 = Select(t=w353, s=w352, f=w351) -> (s? t:f=w348:T2)
      n167 = Equal?(x=w332, y=w350) -> (x = y?=w349:bool)
      n168 = Select(t=w350, s=w349, f=w348) -> (s? t:f=w345:T2)
      n169 = Equal?(x=w332, y=w347) -> (x = y?=w346:bool)
      n170 = Select(t=w347, s=w346, f=w345) -> (s? t:f=w342:T2)
      n171 = Equal?(x=w332, y=w344) -> (x = y?=w343:bool)
      n172 = Select(t=w344, s=w343, f=w342) -> (s? t:f=w339:T2)
      n173 = Equal?(x=w332, y=w341) -> (x = y?=w340:bool)
      n174 = Select(t=w341, s=w340, f=w339) -> (s? t:f=w336:T2)
      n175 = Equal?(x=w332, y=w338) -> (x = y?=w337:bool)
      n176 = Select(t=w338, s=w337, f=w336) -> (s? t:f=w333:T2)
      n177 = Add(x=w321, y=w322) -> (x+y=w320:dbl)
      n178 = Subtract(x=w321, y=w322) -> (x-y=w319:dbl)
      n179 = Equal?(x=w332, y=w335) -> (x = y?=w334:bool)
      n180 = In Range and Coerce(upper limit=w320, x=w325, lower limit=w319) -> (In Range?=w327:bool)  [unwired: 1 out]
      n181 = Select(t=w335, s=w334, f=w333) -> (s? t:f=w331:T2)
      n182 = Not(x=w327) -> (.not. x?=w326:bool)
      n183 = Select(t=TRUE, s=w326, f=FALSE) -> (s? t:f=w324:bool)
    }
    frame "Cargo High" {
      w360 = TRUE
      w364 = 150.0
      w361 = 50000.0
      w377 = T2."Cargo High" ("Lift State")
      w380 = T2."Cargo Feed" ("Lift State")
      w383 = T2."Cargo Ship" ("Lift State")
      w386 = T2."Hatch Low" ("Lift State")
      w389 = T2."Cargo Mid" ("Lift State")
      w392 = T2."Cargo Low" ("Lift State")
      w395 = T2."Hatch High" ("Lift State")
      w398 = T2."Hatch Mid" ("Lift State")
      w399 = T2."Ground" ("Lift State")
      # "Was Originally 50000"
      n184 = Equal?(x=w374, y=w399) -> (x = y?=w400:bool)
      n185 = Select(t=w399, s=w400, f=T2."Cargo High" ("Lift State")) -> (s? t:f=w396:T2)
      n186 = Equal?(x=w374, y=w398) -> (x = y?=w397:bool)
      n187 = Select(t=w398, s=w397, f=w396) -> (s? t:f=w393:T2)
      n188 = Equal?(x=w374, y=w395) -> (x = y?=w394:bool)
      n189 = Select(t=w395, s=w394, f=w393) -> (s? t:f=w390:T2)
      n190 = Equal?(x=w374, y=w392) -> (x = y?=w391:bool)
      n191 = Select(t=w392, s=w391, f=w390) -> (s? t:f=w387:T2)
      n192 = Equal?(x=w374, y=w389) -> (x = y?=w388:bool)
      n193 = Select(t=w389, s=w388, f=w387) -> (s? t:f=w384:T2)
      n194 = Equal?(x=w374, y=w386) -> (x = y?=w385:bool)
      n195 = Select(t=w386, s=w385, f=w384) -> (s? t:f=w381:T2)
      n196 = Equal?(x=w374, y=w383) -> (x = y?=w382:bool)
      n197 = Select(t=w383, s=w382, f=w381) -> (s? t:f=w378:T2)
      n198 = Equal?(x=w374, y=w380) -> (x = y?=w379:bool)
      n199 = Add(x=w361, y=w364) -> (x+y=w362:dbl)
      n200 = Subtract(x=w361, y=w364) -> (x-y=w363:dbl)
      n201 = Select(t=w380, s=w379, f=w378) -> (s? t:f=w375:T2)
      n202 = Equal?(x=w374, y=w377) -> (x = y?=w376:bool)
      n203 = In Range and Coerce(upper limit=w362, x=w365, lower limit=w363) -> (In Range?=w369:bool)  [unwired: 1 out]
      n204 = Select(t=w377, s=w376, f=w375) -> (s? t:f=w373:T2)
      n205 = Not(x=w369) -> (.not. x?=w368:bool)
      n206 = Select(t=TRUE, s=w368, f=FALSE) -> (s? t:f=w366:bool)
    }
    frame "Cargo Ship" {
      w402 = FALSE
      w406 = 150.0
      w405 = 30000.0
      w419 = T2."Cargo Ship" ("Lift State")
      w422 = T2."Cargo Feed" ("Lift State")
      w425 = T2."Hatch Low" ("Lift State")
      w428 = T2."Cargo High" ("Lift State")
      w431 = T2."Cargo Mid" ("Lift State")
      w434 = T2."Cargo Low" ("Lift State")
      w437 = T2."Hatch High" ("Lift State")
      w440 = T2."Hatch Mid" ("Lift State")
      w441 = T2."Ground" ("Lift State")
      n207 = Equal?(x=w416, y=w441) -> (x = y?=w442:bool)
      n208 = Select(t=w441, s=w442, f=T2."Cargo Ship" ("Lift State")) -> (s? t:f=w438:T2)
      n209 = Equal?(x=w416, y=w440) -> (x = y?=w439:bool)
      n210 = Select(t=w440, s=w439, f=w438) -> (s? t:f=w435:T2)
      n211 = Equal?(x=w416, y=w437) -> (x = y?=w436:bool)
      n212 = Select(t=w437, s=w436, f=w435) -> (s? t:f=w432:T2)
      n213 = Equal?(x=w416, y=w434) -> (x = y?=w433:bool)
      n214 = Select(t=w434, s=w433, f=w432) -> (s? t:f=w429:T2)
      n215 = Equal?(x=w416, y=w431) -> (x = y?=w430:bool)
      n216 = Select(t=w431, s=w430, f=w429) -> (s? t:f=w426:T2)
      n217 = Equal?(x=w416, y=w428) -> (x = y?=w427:bool)
      n218 = Select(t=w428, s=w427, f=w426) -> (s? t:f=w423:T2)
      n219 = Equal?(x=w416, y=w425) -> (x = y?=w424:bool)
      n220 = Select(t=w425, s=w424, f=w423) -> (s? t:f=w420:T2)
      n221 = Equal?(x=w416, y=w422) -> (x = y?=w421:bool)
      n222 = Select(t=w422, s=w421, f=w420) -> (s? t:f=w417:T2)
      n223 = Equal?(x=w416, y=w419) -> (x = y?=w418:bool)
      n224 = Add(x=w405, y=w406) -> (x+y=w403:dbl)
      n225 = Subtract(x=w405, y=w406) -> (x-y=w404:dbl)
      n226 = Select(t=w419, s=w418, f=w417) -> (s? t:f=w415:T2)
      n227 = In Range and Coerce(upper limit=w403, x=w407, lower limit=w404) -> (In Range?=w412:bool)  [unwired: 1 out]
      n228 = Not(x=w412) -> (.not. x?=w411:bool)
      n229 = Select(t=TRUE, s=w411, f=FALSE) -> (s? t:f=w408:bool)
    }
    frame "Cargo Feed" {
      w444 = FALSE
      w448 = 150.0
      w445 = 50.0
      w461 = T2."Cargo Feed" ("Lift State")
      w464 = T2."Ground" ("Lift State")
      w467 = T2."Cargo Ship" ("Lift State")
      w470 = T2."Cargo High" ("Lift State")
      w473 = T2."Cargo Mid" ("Lift State")
      w476 = T2."Cargo Low" ("Lift State")
      w479 = T2."Hatch High" ("Lift State")
      w482 = T2."Hatch Mid" ("Lift State")
      w483 = T2."Hatch Low" ("Lift State")
      n230 = Equal?(x=w458, y=w483) -> (x = y?=w484:bool)
      n231 = Select(t=w483, s=w484, f=T2."Cargo Feed" ("Lift State")) -> (s? t:f=w480:T2)
      n232 = Equal?(x=w458, y=w482) -> (x = y?=w481:bool)
      n233 = Select(t=w482, s=w481, f=w480) -> (s? t:f=w477:T2)
      n234 = Equal?(x=w458, y=w479) -> (x = y?=w478:bool)
      n235 = Select(t=w479, s=w478, f=w477) -> (s? t:f=w474:T2)
      n236 = Equal?(x=w458, y=w476) -> (x = y?=w475:bool)
      n237 = Select(t=w476, s=w475, f=w474) -> (s? t:f=w471:T2)
      n238 = Equal?(x=w458, y=w473) -> (x = y?=w472:bool)
      n239 = Select(t=w473, s=w472, f=w471) -> (s? t:f=w468:T2)
      n240 = Equal?(x=w458, y=w470) -> (x = y?=w469:bool)
      n241 = Select(t=w470, s=w469, f=w468) -> (s? t:f=w465:T2)
      n242 = Equal?(x=w458, y=w467) -> (x = y?=w466:bool)
      n243 = Select(t=w467, s=w466, f=w465) -> (s? t:f=w462:T2)
      n244 = Equal?(x=w458, y=w464) -> (x = y?=w463:bool)
      n245 = Select(t=w464, s=w463, f=w462) -> (s? t:f=w459:T2)
      n246 = Equal?(x=w458, y=w461) -> (x = y?=w460:bool)
      n247 = Select(t=w461, s=w460, f=w459) -> (s? t:f=w457:T2)
      n248 = Add(x=w445, y=w448) -> (x+y=w447:dbl)
      n249 = Subtract(x=w445, y=w448) -> (x-y=w446:dbl)
      n250 = In Range and Coerce(upper limit=w447, x=w452, lower limit=w446) -> (In Range?=w454:bool)  [unwired: 1 out]
      n251 = Not(x=w454) -> (.not. x?=w453:bool)
      n252 = Select(t=TRUE, s=w453, f=FALSE) -> (s? t:f=w449:bool)
    }
  }
  n253 = Not(x="Calibrate Lift") -> (.not. x?=w3:bool)
  n254 = And(x=w4, y=w3) -> (x .and. y?=w1:bool)
  n255 = Select(t=enum16{"Motion Magic", "Manual", "Disable"}."Disable", s=w1, f=enum16{"Motion Magic", "Manual", "Disable"}."Motion Magic" ("t")) -> (s? t:f=w17:enum16{"Motion Magic", "Manual", "Disable"})
  n256 = Select(t=enum16{"Motion Magic", "Manual", "Disable"}."Manual", s=w14, f=w17) -> (s? t:f=w16:enum16{"Motion Magic", "Manual", "Disable"})
  n257 = case shown="\"Motion Magic\", Default" w16 {
    tunnel: w31 -> [w490 w498 w500]
    tunnel: "Calibrate Lift" -> [w486 _ _]
    frame "Motion Magic", Default {
      w491 = T12 7 items=["PercentOutput"=0, "Position"=1, "Velocity"=2, "Current"=3, "Follower"=5, "MotionProfile"=6, "MotionMagic"=7, "MotionProfileArc"=10, "Disabled"=15] ("Control Mode")
      n258 = local read "Setpoint"() -> (w489:dbl)
      n259 = Select(t="Lift Setpoint", s=w486, f=w489) -> (s? t:f=w488:dbl)
      n260 = call <vilib>:"CTRE_Phoenix_MotorControl_Set.vi"("Output"=w488, "Control Mode"=w491, "PhoenixMotorControlDevRef"=w490) -> ()  [unwired: 7 in, 2 out]
    }
    frame "Manual" {
      w497 = T12 0 items=["PercentOutput"=0, "Position"=1, "Velocity"=2, "Current"=3, "Follower"=5, "MotionProfile"=6, "MotionMagic"=7, "MotionProfileArc"=10, "Disabled"=15] ("Control Mode")
      n261 = call-poly <vilib>:"NT Read Value.vi"("Name"="Manual Lift Control") -> ("Numeric"=w493:dbl)  [unwired: 9 in, 1 out]
      n262 = Select(t="Output", s="Enable Manual", f=w493) -> (s? t:f=w495:dbl)
      n263 = call <vilib>:"CTRE_Phoenix_MotorControl_Set.vi"("Output"=w495, "Control Mode"=w497, "PhoenixMotorControlDevRef"=w498) -> ()  [unwired: 7 in, 2 out]
    }
    frame "Disable" {
      w501 = T12 0 items=["PercentOutput"=0, "Position"=1, "Velocity"=2, "Current"=3, "Follower"=5, "MotionProfile"=6, "MotionMagic"=7, "MotionProfileArc"=10, "Disabled"=15] ("Control Mode")
      n264 = call <vilib>:"CTRE_Phoenix_MotorControl_Set.vi"("Output"=0.0, "Control Mode"=w501, "PhoenixMotorControlDevRef"=w500) -> ()  [unwired: 7 in, 2 out]
    }
  }
  n265 = disable-structure shown="Disabled" {
    disable-tunnel: [w503 _] -> _
    disable-tunnel: _ -> [w502 _]
    frame Disabled {
      n266 = feedback #1(T2."Idle" ("Lift State")) -> (w503:T2)
      n267 = feedback-in #1(w502) -> ()
    }
    frame Enabled {
    }
  }
  n268 = local write "reset pos"(w23) -> ()
  n269 = local write "Disable?"(w26) -> ()
  n270 = disable-structure shown="Disabled" {
    frame Disabled {
      n271 = global read "Robot Global Data.vi" "Lift State"() -> ()  [unwired: 1 in]
    }
    frame Enabled {
    }
  }
  n272 = local write "Lift Shift"(TRUE ("Lift Shift")) -> ()
  n273 = global write "Robot Global Data.vi" "Cargo High"(w7) -> ()
  n274 = global write "Robot Global Data.vi" "Cargo Mid"(w6) -> ()
  n275 = global write "Robot Global Data.vi" "Cargo Low"(w5) -> ()
  n276 = local write "Setpoint"(w25) -> ()
